vi "SCANNER.vi"() -> ()   [LabVIEW 2025]
panel:
  out "error out":errorcluster
  out "listener address list":i16[](array[numeric])
  out "Instruments":string[](array[string])
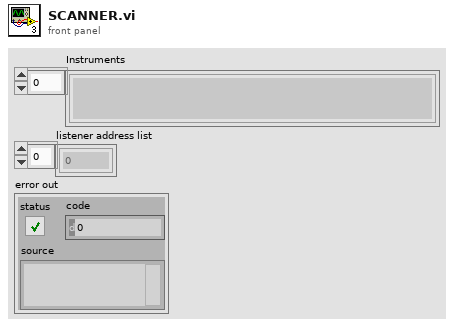
[diagram p1: front panel]
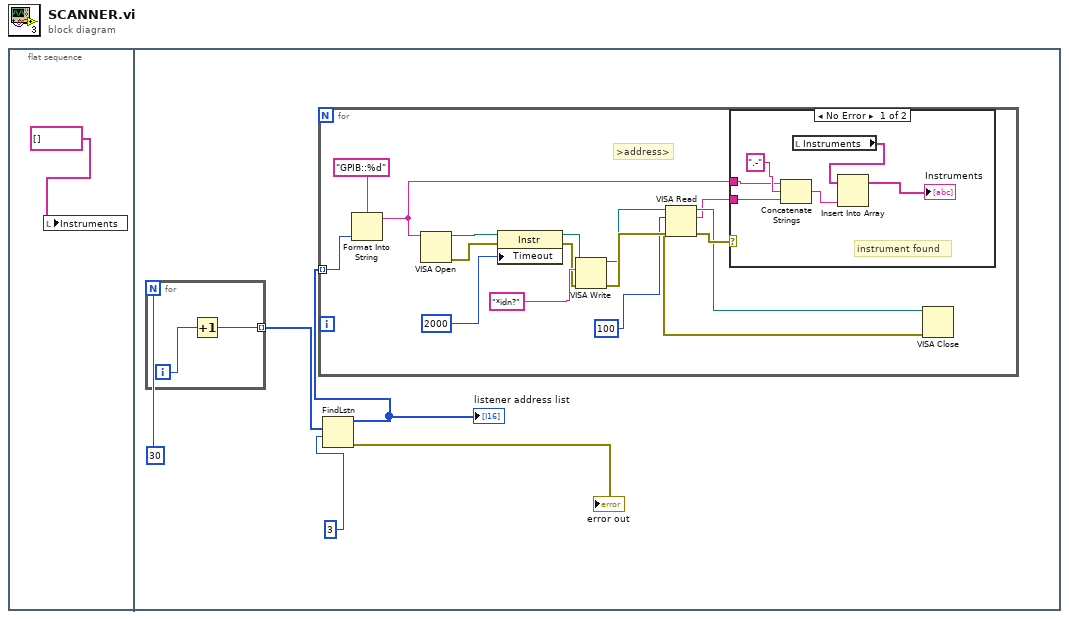
[diagram p0: block diagram]
diagram:
  n1 = flat-sequence {
    frame #0 {
      n2 = local write "Instruments"(string[] []) -> ()
    }
    frame #1 {
      n3 = for {
        N: 30 -> [_]
        tunnel: [w7] -> w5 mode=indexing
        i -> [w8]
        n4 = Increment(x=w8) -> (x+1=w7:i32)
      }
      n5 = FindLstn(5:3, 6:w5) -> (0:→"error out":errorcluster, 3:w2:i16[])  [unwired: 2 in, 2 out]
      "listener address list" <- w2
      n6 = for {
        tunnel: w2 -> [w9] mode=indexing
        # ">address>"
        n7 = Format Into String(format string="GPIB::%d", w9) -> (resulting string=w22:string)  [unwired: 2 in, 1 out]
        n8 = VISA Open(VISA resource name=w22) -> (VISA resource name=w21:refnum<visa-resource-name>, error out=w20:errorcluster)  [unwired: 4 in]
        n9 = property class="Instr"(reference=w21, error in=w20, "Timeout"=2000) -> (reference out=w19:refnum<visa-resource-name>, error out=w17:errorcluster)
        n10 = VISA Write(VISA resource name=w19, write buffer="*idn?", error in (no error)=w17) -> (VISA resource name out=w14:refnum<visa-resource-name>, error out=w16:errorcluster)  [unwired: 1 out]
        n11 = VISA Read(VISA resource name=w14, byte count=100, error in (no error)=w16) -> (VISA resource name out=w13:refnum<visa-resource-name>, read buffer=w12:string, error out=w15:errorcluster)  [unwired: 1 out]
        n12 = case shown="No Error" w15 {
          tunnel: w22 -> [w26 _]
          tunnel: w12 -> [w25 _]
          frame No Error {
            # "instrument found"
            n13 = Concatenate Strings(w26, ".-", w25) -> (w28:string)
            n14 = local read "Instruments"() -> (w24:string[])
            n15 = Insert Into Array(array=w24, new element=w28) -> (→"Instruments":string[])  [unwired: 1 in]
          }
          frame Error {
          }
        }
        n16 = VISA Close(VISA resource name=w13, error in (no error)=w15) -> ()  [unwired: 1 out]
      }
    }
  }
